vi "Control Panel.vi"(8 "error in (no error)":errorcluster, 11 "Control Panel":T1) -> (0 "error out":errorcluster, 1 "VPI":bool, 2 "DVA":bool, 3 "E-CAL":bool, 4 "VSA":bool, 5 "HD/CYC":bool, 6 "HS":bool, 7 "Verify Socket":bool)   [LabVIEW 2012]
panel:
  # "Indicator"
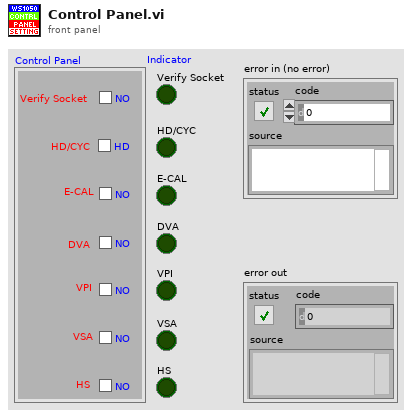
[diagram p1: front panel]
types:
  T1 = cluster{"Verify Socket":bool, "HD/CYC":bool, "E-CAL":bool, "DVA":bool, "VPI":bool, "VSA":bool, "HS":bool}
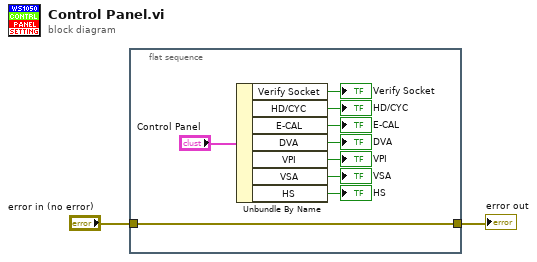
[diagram p0: block diagram]
diagram:
  n1 = flat-sequence {
    tunnel: "error in (no error)" -> [w3]
    tunnel: [w3] -> w1
    frame #0 {
      n2 = Unbundle By Name("Control Panel") -> ("Verify Socket"=→"Verify Socket":bool, "HD/CYC"=→"HD/CYC":bool, "E-CAL"=→"E-CAL":bool, "DVA"=→"DVA":bool, "VPI"=→"VPI":bool, "VSA"=→"VSA":bool, "HS"=→"HS":bool)
    }
  }
  "error out" <- w1
